vi "GUI_IP2_DPM.vi"() -> ()   [LabVIEW 2020]
uses:
  Shared/GUI_Template/GUI_master/tcp new data cluster.ctl
panel:
  in  "Array Y":dbl[](array[numeric])
  in  "Array X":dbl[](array[numeric])
  out "XY Graph":cluster{dbl[], dbl[]}(graph)
  in  "Clear":bool
  in  "Plot":bool
  in  "gain::2":dbl=0.01 caption="gain" min=0.0 max=240.0
  in  "gain::3":dbl=0.01 caption="gain" min=0.0 max=40.0
  in  "exposure::2":dbl=0.01 caption="exposure" min=3.8e-05 max=1.0
  in  "Position.Channel 4::5":i16 caption="PM1 CAM block\n20 =Out | 0=In" min=0 max=40
  in  "Position.Channel 1::5":i16 caption="PM1 align\n39=mirror | 70=dump" min=0 max=40
  in  "Position.device 2::4":i64 caption="PM2 Horizontal" min=-10000000 max=10000000
  in  "Position.device 4::4":i64 caption="PM1 Vertical" min=-10000000 max=10000000
  in  "Position.device 3::4":i64 caption="PM1 Horizontal" min=-10000000 max=10000000
  in  "Position.device 1::4":i64 caption="PM2 Vertical" min=-10000000 max=10000000
  in  "Position.Stage A::1":dbl caption="DPM-X" min=0.0 max=300.0
  in  "Position.Stage C::1":dbl caption="DPM-Z" min=0.0 max=100.0
  in  "GUIdevice 5":string="STAGE-PL1-Smaract"
  in  "GUIdevice 4":string="MCD-PL1-picosOFI1"
  in  "exposure::3":dbl=0.01 caption="exposure" min=3.8e-05 max=1.0
  out "image::3":T1(plugin-control) caption="CAM-PL1-LPMode"
  in  "GUIdevice 3":string="CAM-PL1-LPMode"
  out "image::2":T1(plugin-control) caption="CAM-PL1-SideSpec"
  in  "GUIdevice 2":string="CAM-PL1-SideSpec"
  in  "Motor status::1":string caption="DPM Stage"
  in  "Position.Stage B::1":dbl caption="DPM-Y" min=0.0 max=105.0
  out "device status::1":string="Initialized"
  in  "stop":bool
  in  "GUIdevice 1":string="MCD-PL1-NewmarkDPM"
  # "PM1 CAM"
  # "Z"
  # "X"
  # "Y"
  # "PM2 CAM"
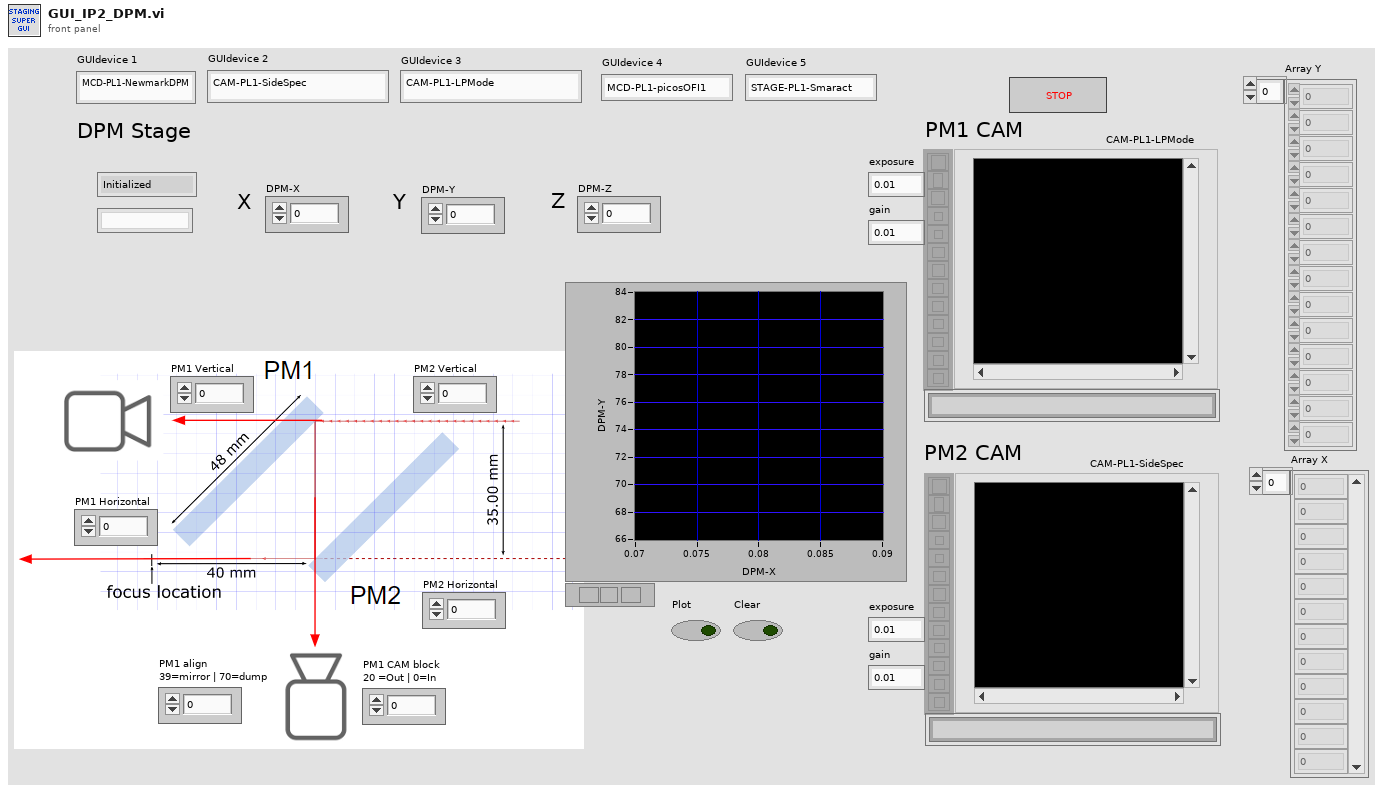
[diagram p1: front panel]
types:
  T1 = typedef "IMAQ Image.ctl" = refnum<image>
  T2 = typedef "Image Type" = u32
  T3 = typedef "tcp new data cluster.ctl" = cluster{"EventEnum":enum16{"new data", "connection status update"}, "Device name":string}
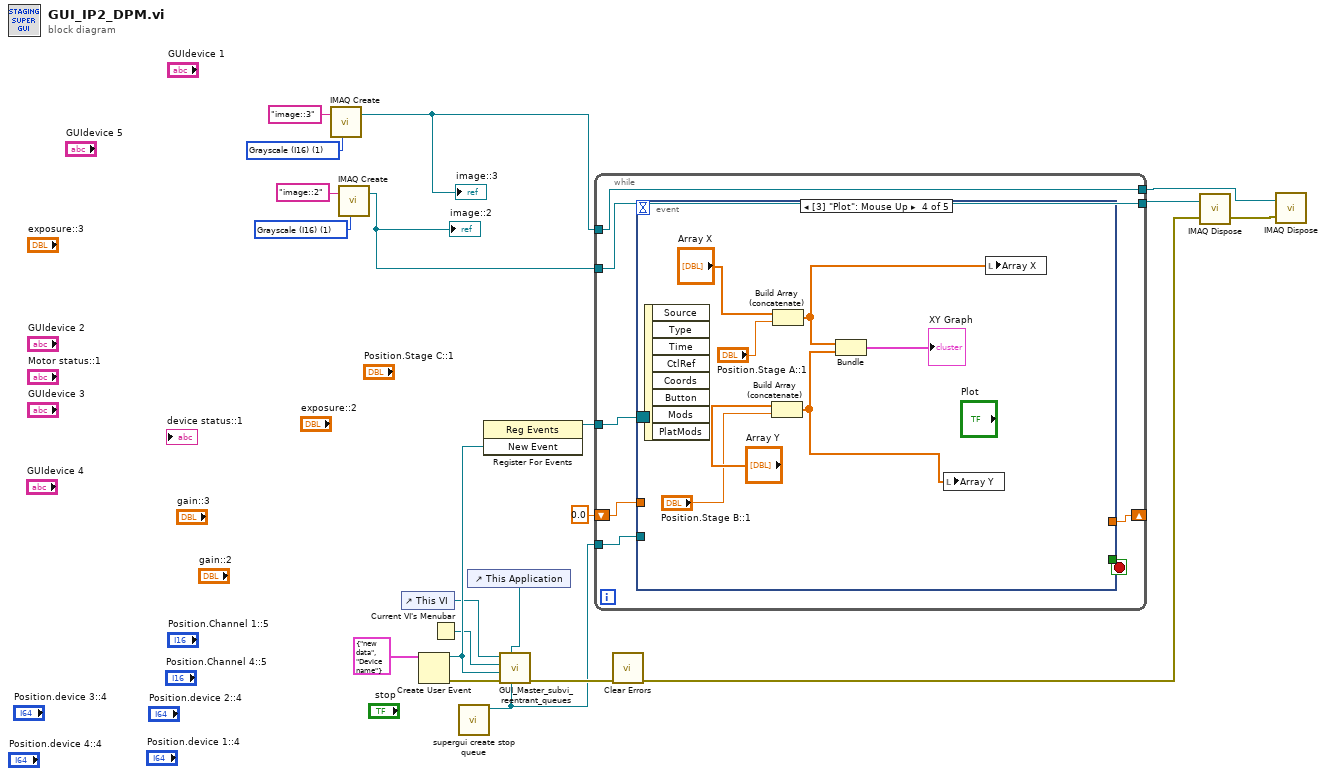
[diagram p0: block diagram]
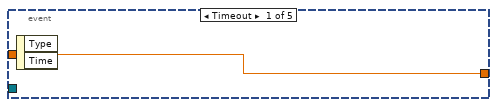
[diagram p2: hidden frame]
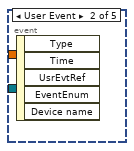
[diagram p3: hidden frame]
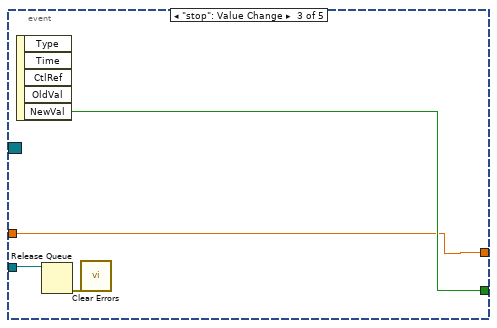
[diagram p4: hidden frame]
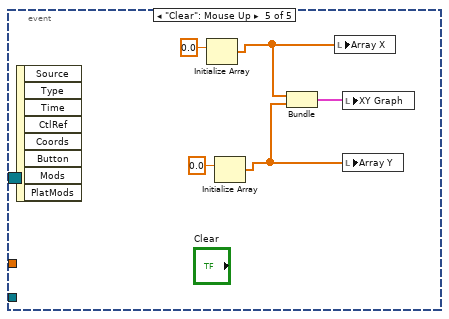
[diagram p5: hidden frame]
diagram:
  w9 = T2 1 items=["Grayscale (U8)", "Grayscale (I16)", "Grayscale (SGL)", "Complex (CSG)", "RGB (U32)", "HSL (U32)", "RGB (U64)", "Grayscale (U16)"] ("Image Type")
  w13 = T2 1 items=["Grayscale (U8)", "Grayscale (I16)", "Grayscale (SGL)", "Complex (CSG)", "RGB (U32)", "HSL (U32)", "RGB (U64)", "Grayscale (U16)"] ("Image Type")
  n1 = call "IMAQ Create"("Image Name"="image::3", "Image Type"=w9) -> ("New Image"=w7:T1)  [unwired: 3 in, 1 out]
  "image::3" <- w7
  n2 = call "IMAQ Create"("Image Name"="image::2", "Image Type"=w13) -> ("New Image"=w12:T1)  [unwired: 3 in, 1 out]
  "image::2" <- w12
  n3 = control-ref of="This VI"() -> (w4:refnum<vi>)
  n4 = Create User Event(user event datatype=T3 {"EventEnum"=enum."new data", "Device name"="Device name"} ("New Event")) -> (user event=w17:refnum<user-event>, error out=w19:errorcluster)  [unwired: 1 in]
  n5 = Current VI's Menubar() -> (w3:refnum<k9>)
  n6 = call "supergui create stop queue.vi"() -> ("STOP Queue out"=w1:refnum<queue>)  [unwired: 11 in]
  n7 = control-ref of="This Application"() -> (w2:refnum<vi>)
  n8 = register-events(w17) -> (reference out=w16:refnum<event-registration>)  [unwired: 2 in, 1 out]
  n9 = call "GUI_Master_subvi_reentrant_queues.vi"("STOP Queue in"=w1, "This Application"=w2, "error in (no error)"=w19, "tcp data event"=w17, "Caller menu reference"=w3, "Caller VI ref"=w4) -> ("error out"=w18:errorcluster)  [unwired: 5 in]
  n10 = while {
    tunnel: w16 -> [w27]
    shift-right: [w24] -> _
    shift-left: 0.0 -> [w25]
    tunnel: w12 -> [w23]
    tunnel: [w23] -> w11
    tunnel: w7 -> [w22]
    tunnel: [w22] -> w5
    tunnel: w1 -> [w21]
    stop <- w26 stop-if-true
    n11 = event shown="[3] \"Plot\": Mouse Up" {
      selector: w27 -> [_ _ _ _ _]
      dyn-events: _ -> [_ _ _ _ _]
      timeout: _ -> [_ _ _ _ _]
      tunnel: [_ _ w32 _ _] -> w26
      tunnel: w25 -> [w28 _ w31 _ _]
      tunnel: [w28 _ w31 _ _] -> w24
      tunnel: w21 -> [_ _ w30 _ _]
      event Timeout {
        n12 = event-data() -> ()  [unwired: 1 in, 2 out]
      }
      event User Event {
        n13 = event-data() -> ()  [unwired: 1 in, 5 out]
      }
      event "stop": Value Change {
        n14 = event-data() -> ("NewVal"=w32:bool)  [unwired: 1 in, 4 out]
        n15 = Release Queue(queue=w30) -> (error out=w29:errorcluster)  [unwired: 2 in, 2 out]
        n16 = call <vilib>:"Clear Errors.vi"("error in (no error)"=w29) -> ()  [unwired: 5 in, 2 out]
      }
      event "Plot": Mouse Up {
        n17 = event-data() -> ()  [unwired: 1 in, 8 out]
        n18 = Build Array (concatenate)("Array Y", "Position.Stage B::1") -> (w36:dbl[])
        n19 = Build Array (concatenate)("Array X", "Position.Stage A::1") -> (w35:dbl[])
        n20 = Bundle(w35, w36) -> (→"XY Graph":cluster{dbl[], dbl[]})  [unwired: 1 in]
        n21 = local write "Array Y"(w36) -> ()
        n22 = local write "Array X"(w35) -> ()
      }
      event "Clear": Mouse Up {
        n23 = event-data() -> ()  [unwired: 1 in, 8 out]
        n24 = Initialize Array(0.0 ("element")) -> (w41:dbl[])  [unwired: 1 in]
        n25 = Initialize Array(0.0 ("element")) -> (w42:dbl[])  [unwired: 1 in]
        n26 = Bundle(w41, w42) -> (w40:cluster{dbl[], dbl[]})  [unwired: 1 in]
        n27 = local write "Array X"(w41) -> ()
        n28 = local write "XY Graph"(w40) -> ()
        n29 = local write "Array Y"(w42) -> ()
      }
    }
  }
  n30 = call <vilib>:"Clear Errors.vi"("error in (no error)"=w18) -> ("error out"=w10:errorcluster)  [unwired: 5 in, 1 out]
  n31 = call "IMAQ Dispose"("Image"=w11, "error in (no error)"=w10) -> ("error out"=w6:errorcluster)  [unwired: 4 in]
  n32 = call "IMAQ Dispose"("Image"=w5, "error in (no error)"=w6) -> ()  [unwired: 4 in, 1 out]
